vi "Set Border.vi"(8 "error in (no error)":errorcluster, 10 "Scalable Border.lvclass":refnum<class "Scalable Border.lvclass">, 11 "Graphic in":refnum<class "Graphic.lvclass">) -> (0 "error out":errorcluster, 3 "Graphic out":refnum<class "Graphic.lvclass">)   [LabVIEW 2015, in "Graphic.lvclass"]
uses:
  Graphic.lvclass
  Scalable Border/Scalable Border.lvclass
  Graphic.lvclass/Graphic.ctl
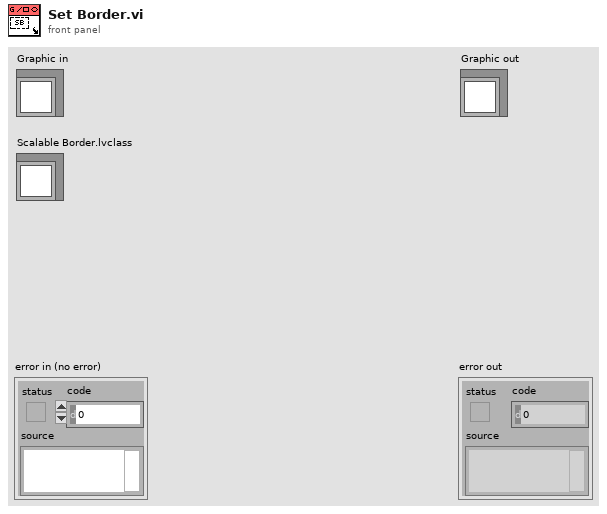
[diagram p1: front panel]
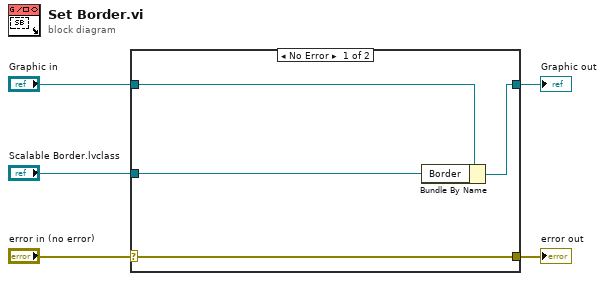
[diagram p0: block diagram]
diagram:
  n1 = case shown="No Error" "error in (no error)" {
    selector: "error in (no error)" -> [w9 w10]
    tunnel: [w9 w10] -> w4
    tunnel: [w7 w11] -> w2
    tunnel: "Graphic in" -> [w8 w11]
    tunnel: "Scalable Border.lvclass" -> [w6 _]
    frame No Error {
      n2 = Bundle By Name(cluster=w8, "Border"=w6) -> (w7:refnum<class "Graphic.lvclass">)
    }
    frame Error {
    }
  }
  "error out" <- w4
  "Graphic out" <- w2
